vi "Load and Save Controls.vi"(4 "path":path, 6 "Use vi Path":bool, 8 "error in (no error)":errorcluster, 11 "Control References":refnum<vi>[](array[refnum])) -> (0 "error out":errorcluster)   [LabVIEW 2018]
uses:
  RWC_Actions.ctl
panel:
  out "ctrl file path out":path
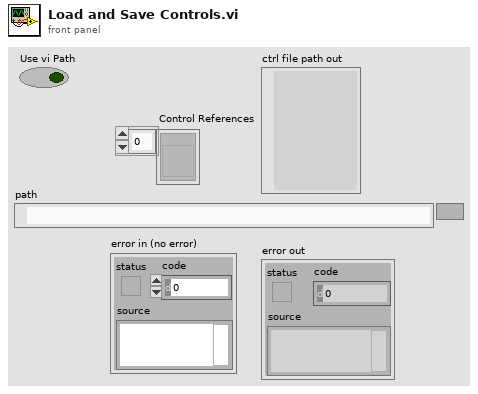
[diagram p1: front panel]
types:
  T1 = typedef "RWC_Actions.ctl" = enum16{"Read", "Write", "Read and Create"}
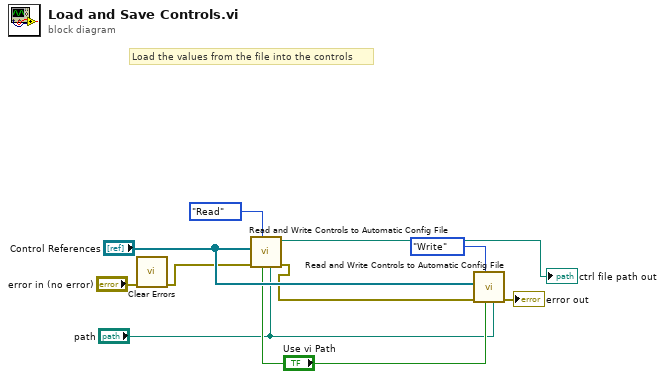
[diagram p0: block diagram]
diagram:
  # "Load the values from the file into the controls"
  n1 = call <vilib>:"Clear Errors.vi"("error in (no error)"="error in (no error)") -> ("error out"=w7:errorcluster)  [unwired: 5 in, 1 out]
  n2 = call "Read and Write Controls to Automatic Config File.vi"("path"="path", "Use Path"="Use vi Path", "Action"=RWC_Actions."Read", "error in"=w7, "Control References"="Control References") -> ("error out"=w8:errorcluster, "ctrl file path"=→"ctrl file path out":path)  [unwired: 5 in]
  n3 = call "Read and Write Controls to Automatic Config File.vi"("path"="path", "Use Path"="Use vi Path", "Action"=RWC_Actions."Write", "error in"=w8, "Control References"="Control References") -> ("error out"=→"error out":errorcluster)  [unwired: 5 in, 1 out]
